vi "Main_24A.vi"() -> ()   [LabVIEW 2024]
uses:
  Cluster_Function.ctl
  ENUM_Operand.ctl
  <vilib>/Utility/error.llb/Trim Whitespace One-Sided.vi
panel:
  out "Answer Array":bool[](array[boolean])
  out "Map Final":map{string, bool}(c390)
  out "Wire Count":i32
  out "Array":T1[](array[typedef])
  out "Map Start":map{string, bool}(c390)
  in  "Select Data":enum32{"Example", "Example 2", "Puzzle"}(tab)
  in  "Example":string="x00: 1\nx01: 1\nx02: 1\ny00: 0\ny01: 1\ny02: 0\n\nx00 AND y00 -> z00\nx01 XOR y01 -> z01\nx02 OR y02 -> z02"
  in  "Example 2":string="x00: 1\nx01: 0\nx02: 1\nx03: 1\nx04: 0\ny00: 1\ny01: 1\ny02: 1\ny03: 1\ny04: 1\n\nntg XOR fgs -> mjb\ny02 OR x01 -> tnw\nkwq OR kpj -> z05\nx00 OR x03 -> fst\ntgd XOR rvg -> z01\nvdt OR tnw -> bfw\nbfw AND frj -> z10\nffh OR nrd -> bqk\ny00 AND y03 -> djm\ny03 OR y00 -> psh\nbqk OR frj -> z08\ntnw OR fst -> frj\ngnj AND tgd -> z11\nbfw XOR mjb -> z00\nx03 OR x00 -> vdt\ngnj AND wpb -> z02\nx04 AND y00 -> kjc\ndjm OR pbm -> qhw\nnrd AND vdt -> hwm\nkjc AND fst -> rvg\ny04 OR y02 -> fgs\ny01 AND x02 -> pbm\nntg OR kjc -> kwq\npsh XOR fgs -> tgd\nqhw XOR tgd -> z09\npbm OR djm -> kpj\nx03 XOR y03 -> ffh\nx00 XOR y04 -> ntg\nbfw OR bqk -> z06\nnrd XOR fgs -> wpb\nfrj XOR qhw -> z04\nbqk OR frj -> z07\ny03 OR x01 -> nrd\nhwm AND bqk -> z03\ntgd XOR rvg -> z12\ntnw OR pbm -> gnj"
  in  "Puzzle":string="x00: 1\nx01: 0\nx02: 1\nx03: 1\nx04: 0\nx05: 0\nx06: 1\nx07: 1\nx08: 0\nx09: 1\nx10: 1\nx11: 1\nx12: 1\nx13: 1\nx14: 1\nx15: 0\nx16: 1\nx17: 0\nx18: 1\nx19: 1\nx20: 0\nx21: 0\nx22: 1\nx23: 0\nx24: 1\nx25: 0\nx26: 1\nx27: 0\nx28: 1\nx29: 1\nx30: 0\nx31: 0\nx32: 1\nx33: 1\nx34: 1\nx35: 0\nx36: 1\nx37: 1\nx38: 0\nx39: 0\nx40: 1\nx41: 1\nx42: 0\nx43: 0\nx44: 1\ny00: 1\ny01: 0\ny02: 0\ny03: 1\ny04: 1\ny05: 0\ny06: 0\ny07: 0\ny08: 0\ny09: 0\ny10: 0\ny11: 1\ny12: 0\ny13: 0\ny14: 1\ny15: 1\ny16: 0\ny17: 0\ny18: 1\ny19: 0\ny20: 0\ny21: 0\ny22: 1\ny23: 1\ny24: 0\ny25: 0\ny26: 0\ny27: 1\ny28: 1\ny29: 1\ny30: 0\ny31: 1\ny32: 1\ny33: 0\ny34: 1\ny35: 1\ny36: 0\ny37: 0\ny38: 1\ny39: 1\ny40: 1\ny41: 0\ny42: 0\ny43: 1\ny44: 1\n\nnjs AND pvb -> fjh\ny12 AND x12 -> dcm\nsrv XOR dfc -> z22\nqwb XOR vmp -> z14\nnjs XOR pvb -> z10\ncjn OR dfj -> fgc\nkpp XOR tvh -> z34\ntbq OR rdf -> frv\ny40 AND x40 -> drs\npqh XOR mmh -> z05\nx26 XOR y26 -> jkt\nqqp AND dmw -> kqp\nqsh OR wfw -> qcr\nhvw AND qnn -> vgk\nbkc OR wsq -> ckv\nckv XOR bbh -> z03\nfrj XOR hqq -> z02\nqff OR stw -> wsv\nqpq XOR vnr -> z30\npbk XOR kqc -> z15\nmvp OR pbv -> dbj\nx15 AND y15 -> qsh\nwcs OR cqk -> kpp\nbmr XOR fgc -> z32\ny42 XOR x42 -> qjf\nsrv AND dfc -> rng\nrsq AND nts -> brq\nfhv AND hjw -> wwg\nx06 AND y06 -> phw\nvtf AND gdw -> kpc\nwvv AND wbf -> qdh\ny28 AND x28 -> nhs\ny04 AND x04 -> ttv\ncts XOR bcd -> qqp\nmmh AND pqh -> rkt\nhjw XOR fhv -> z37\njdd AND rbm -> z36\ndrt XOR tpt -> z31\ny20 XOR x20 -> gcf\nx27 AND y27 -> ptf\nqnn XOR hvw -> z41\nx13 AND y13 -> msq\ncbr XOR hjd -> z07\nmkv OR hgp -> z45\ny35 XOR x35 -> spp\nx08 XOR y08 -> nrk\ny03 XOR x03 -> bbh\nfhc OR ggh -> fwt\nwhj AND vrh -> qpj\nx34 XOR y34 -> tvh\ny43 AND x43 -> mpm\ny15 XOR x15 -> pbk\nx23 XOR y23 -> bcd\nbwv AND tcd -> sgv\nbcd AND cts -> jcd\nggs OR qmw -> tpt\ngdm XOR jkm -> z09\ny38 XOR x38 -> pgm\nx19 AND y19 -> vmc\ndtc OR ggg -> kqc\nhqq AND frj -> bkc\nsmv OR wwg -> bhh\ny17 AND x17 -> tfq\nx14 AND y14 -> dtc\ny39 AND x39 -> ggh\njmh AND cjc -> gfp\nmgj XOR wsv -> z12\nftd AND wcw -> hjm\ny19 XOR x19 -> whj\nnrk AND ksd -> vwf\nfgq AND spp -> drp\nrsq XOR nts -> z18\ny10 XOR x10 -> njs\nfrv XOR qdb -> z04\nwbk OR fcv -> fgq\nwhj XOR vrh -> z19\ntvh AND kpp -> wbk\ny39 XOR x39 -> pwt\nscg OR gkj -> grv\ndfn XOR qcr -> pbv\nx27 XOR y27 -> ftd\nsvg OR tfq -> rsq\nfkd XOR fwt -> z40\nx07 AND y07 -> pdq\ny13 XOR x13 -> hnt\ngrv XOR vpm -> z21\ny02 XOR x02 -> frj\njkt XOR dbp -> z26\nwdr OR jcd -> z23\nx21 AND y21 -> wns\ny08 AND x08 -> btn\nqqp XOR dmw -> z24\nx01 AND y01 -> wqt\nfrw AND hdp -> hgq\nfrk AND wpk -> hgp\nx07 XOR y07 -> cbr\nx29 AND y29 -> jgm\nsgv OR wqt -> hqq\ntpt AND drt -> dfj\nsdn OR rkt -> kqk\nfrv AND qdb -> vjj\nfjh OR thp -> ncw\ny26 AND x26 -> vvr\nx25 AND y25 -> kcs\nftd XOR wcw -> z27\ntcd XOR bwv -> z01\nbrk XOR kqk -> z06\nx10 AND y10 -> thp\nfrw XOR hdp -> z25\npgm AND bhh -> hsh\nx24 XOR y24 -> dmw\nvmc OR qpj -> bkv\nx44 AND y44 -> mkv\nknh OR vgk -> rps\ndfn AND qcr -> mvp\ntqj OR rng -> cts\ntbb OR wns -> srv\nmsq OR pjj -> vmp\ndrs OR ghn -> hvw\nhsh OR rrb -> rms\ndbj XOR bgt -> z17\nmpm OR kpc -> frk\nbgt AND dbj -> svg\nx40 XOR y40 -> fkd\nx16 AND y16 -> z16\ncbr AND hjd -> dvs\nfsb OR drv -> gdw\ncjc XOR jmh -> z29\npdq OR dvs -> ksd\nrpw OR fbq -> fhv\ny05 XOR x05 -> pqh\nx30 AND y30 -> ggs\nbmb OR drp -> jdd\nhnt XOR fbm -> z13\ny42 AND x42 -> fsb\nqpq AND vnr -> qmw\nx11 XOR y11 -> qff\ngcf AND bkv -> gkj\nwvv XOR wbf -> z28\nx05 AND y05 -> sdn\npqp OR phw -> hjd\njdd XOR rbm -> fbq\nnjt OR kqp -> frw\ny00 XOR x00 -> z00\ny31 AND x31 -> cjn\nx32 XOR y32 -> bmr\nx34 AND y34 -> fcv\ny24 AND x24 -> njt\ny06 XOR x06 -> brk\nx12 XOR y12 -> mgj\nckv AND bbh -> tbq\nrps XOR qjf -> z42\nx33 AND y33 -> cqk\ny09 AND x09 -> nhk\ny33 XOR x33 -> mbp\nx04 XOR y04 -> qdb\nx22 AND y22 -> tqj\ny20 AND x20 -> scg\ny01 XOR x01 -> tcd\nfgc AND bmr -> shp\nmbp XOR pnw -> z33\nfrk XOR wpk -> z44\ny43 XOR x43 -> vtf\nx37 XOR y37 -> hjw\ny03 AND x03 -> rdf\nrms XOR pwt -> z39\nbhh XOR pgm -> z38\nspp XOR fgq -> z35\ny22 XOR x22 -> dfc\nqjf AND rps -> drv\nkcs OR hgq -> dbp\ny29 XOR x29 -> cjc\nx25 XOR y25 -> hdp\nhbq OR dcm -> fbm\nbrk AND kqk -> pqp\nqwb AND vmp -> ggg\ngpb OR shp -> pnw\ny02 AND x02 -> wsq\nptf OR hjm -> wvv\nx18 XOR y18 -> nts\nx23 AND y23 -> wdr\nx09 XOR y09 -> jkm\nx36 AND y36 -> rpw\nx32 AND y32 -> gpb\nmbp AND pnw -> wcs\njgm OR gfp -> qpq\nx11 AND y11 -> qnw\nbkv XOR gcf -> z20\nnhk OR ftf -> pvb\ngdw XOR vtf -> z43\nvjj OR ttv -> mmh\nx41 AND y41 -> knh\nncw XOR qnw -> z11\ny28 XOR x28 -> wbf\ny36 XOR x36 -> rbm\nmgj AND wsv -> hbq\nhnt AND fbm -> pjj\nbrq OR bfd -> vrh\nx17 XOR y17 -> bgt\nksd XOR nrk -> z08\nx38 AND y38 -> rrb\nfwt AND fkd -> ghn\nncw AND qnw -> stw\nx18 AND y18 -> bfd\ny00 AND x00 -> bwv\ngdm AND jkm -> ftf\nrms AND pwt -> fhc\nx16 XOR y16 -> dfn\ny37 AND x37 -> smv\nx35 AND y35 -> bmb\ny30 XOR x30 -> vnr\njkt AND dbp -> dbt\ny41 XOR x41 -> qnn\nx31 XOR y31 -> drt\nqdh OR nhs -> jmh\nvwf OR btn -> gdm\ny44 XOR x44 -> wpk\nx14 XOR y14 -> qwb\nx21 XOR y21 -> vpm\npbk AND kqc -> wfw\nvvr OR dbt -> wcw\ngrv AND vpm -> tbb"
  out "Answer 49430469426918":u64
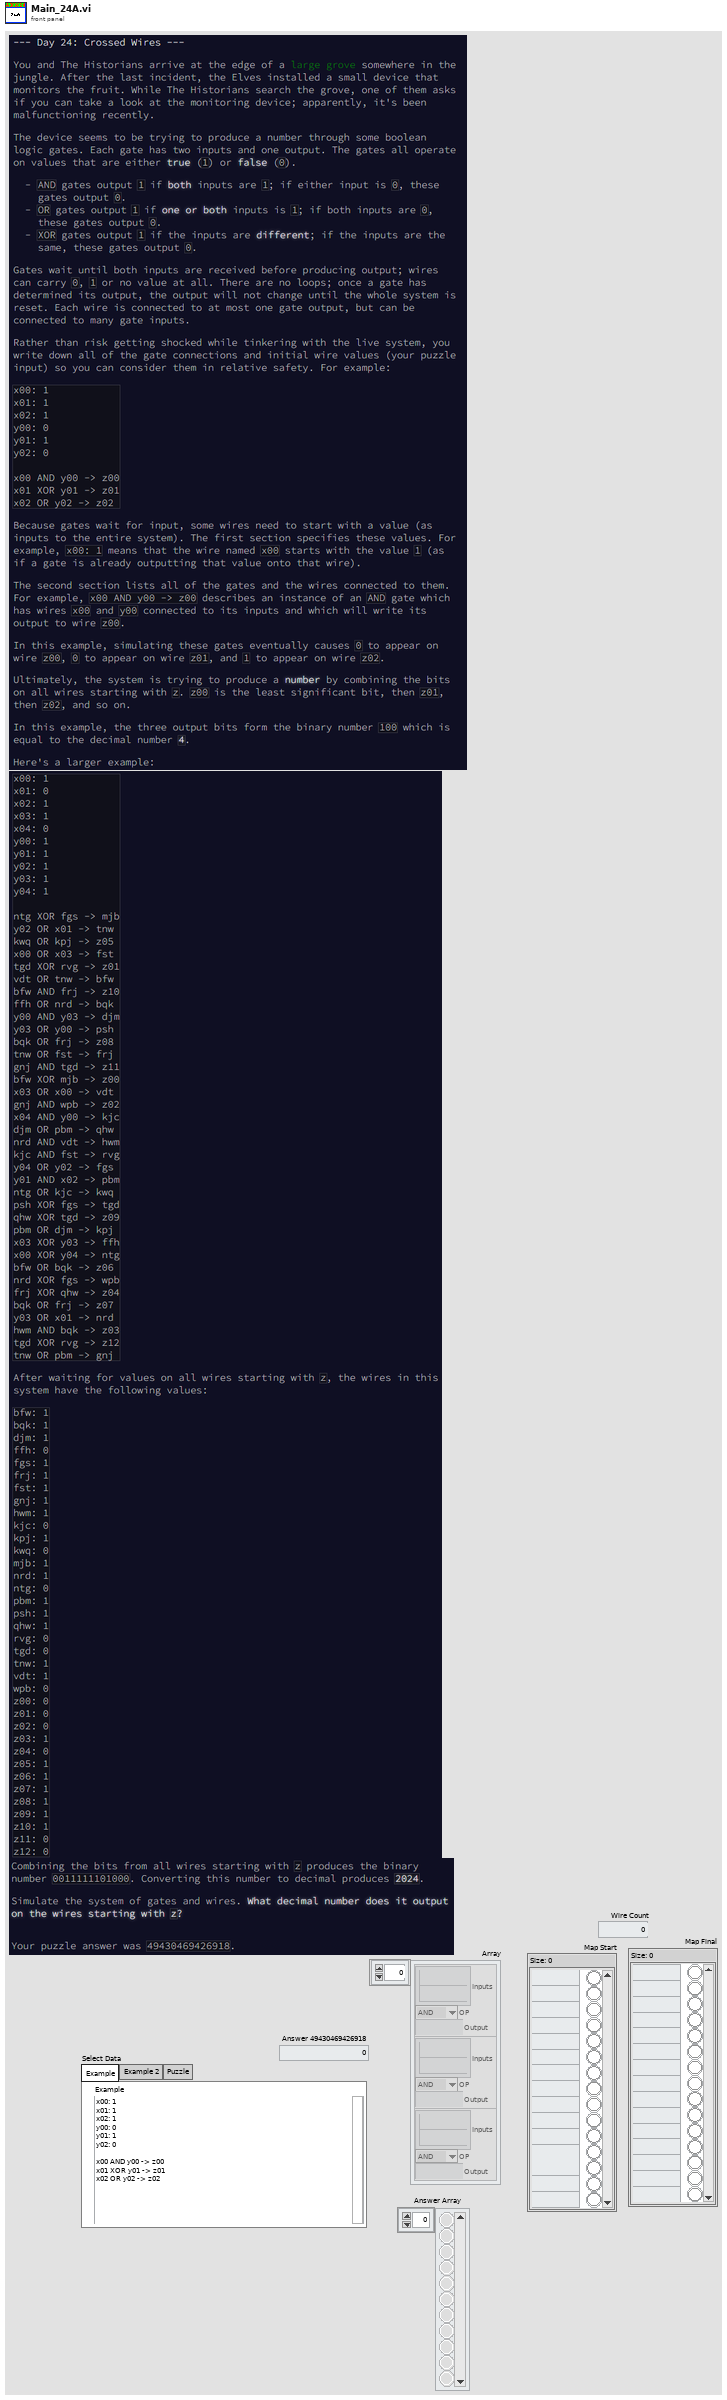
[diagram p1: front panel]
types:
  T1 = typedef "Cluster_Function.ctl" = cluster{"Inputs":string[], "OP":T2, "Output":string}
  T2 = typedef "ENUM_Operand.ctl" = enum16{"AND", "OR", "XOR"}
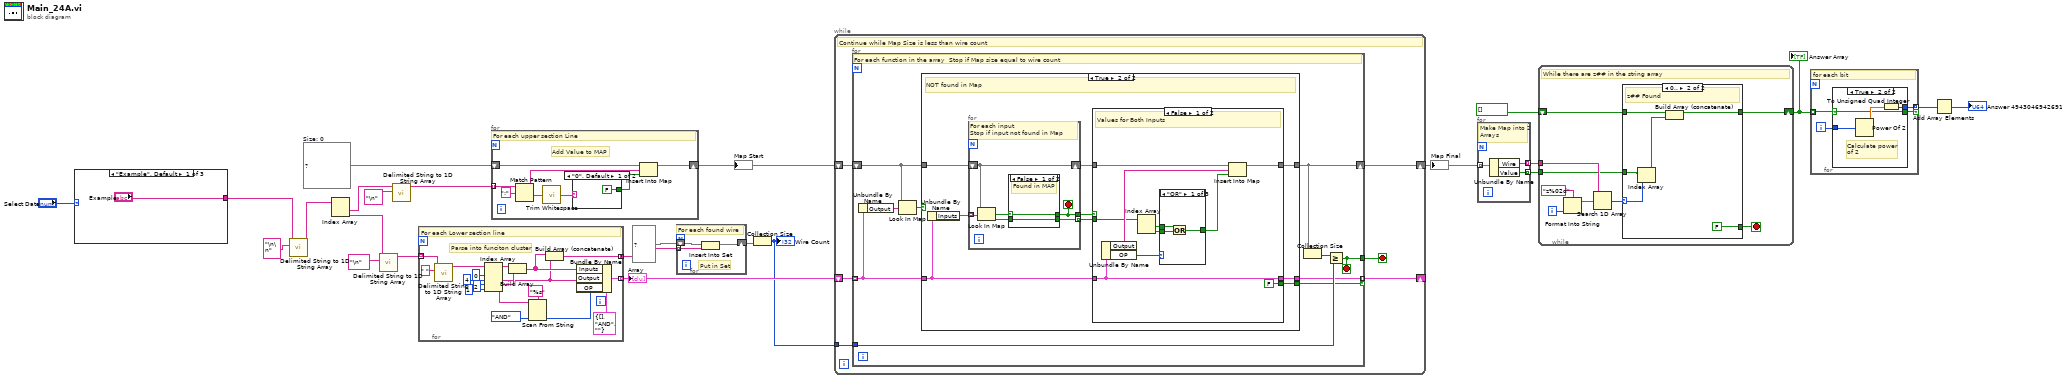
[diagram p0: block diagram]
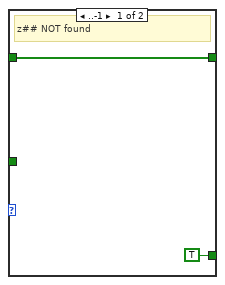
[diagram p3: hidden frame]
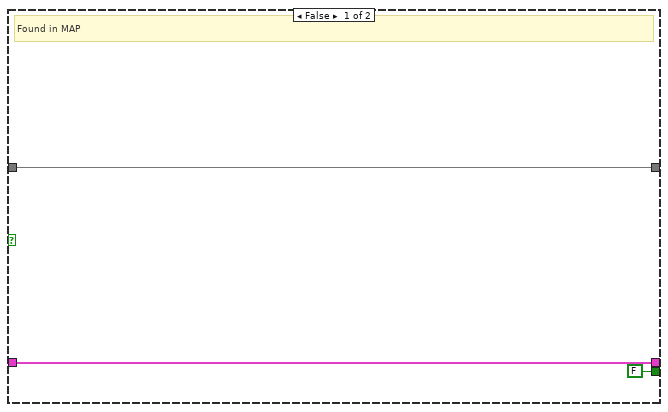
[diagram p4: hidden frame]
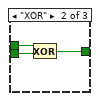
[diagram p5: hidden frame]
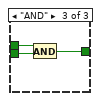
[diagram p6: hidden frame]
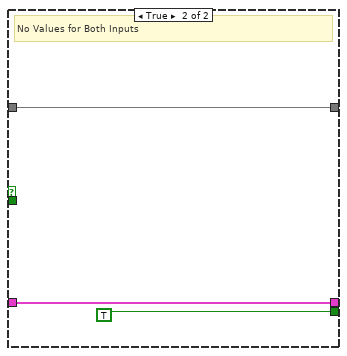
[diagram p7: hidden frame]
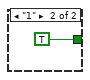
[diagram p9: hidden frame]
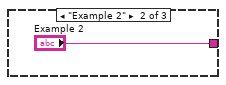
[diagram p10: hidden frame]
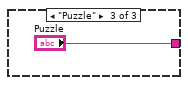
[diagram p11: hidden frame]
diagram:
  w17 = map{string, bool} {}  # Size: 0
  n1 = case shown="\"Example\", Default" "Select Data" {
    tunnel: ["Example" "Example 2" "Puzzle"] -> w22
    frame "Example", Default {
    }
    frame "Example 2" {
    }
    frame "Puzzle" {
    }
  }
  n2 = call <vilib>:"Delimited String to 1D String Array.vi"("delimiter"="\n\n" ("delimiter (Tab)"), "delimited string"=w22) -> ("string array"=w21:string[])  [unwired: 9 in]
  n3 = Index Array(array=w21) -> (element #1=w20:string, element #2=w16:string)  [unwired: 2 in]
  n4 = call <vilib>:"Delimited String to 1D String Array.vi"("delimiter"="\n" ("delimiter (Tab)"), "delimited string"=w16) -> ("string array"=w14:string[])  [unwired: 9 in]
  n5 = call <vilib>:"Delimited String to 1D String Array.vi"("delimiter"="\n" ("delimiter (Tab)"), "delimited string"=w20) -> ("string array"=w18:string[])  [unwired: 9 in]
  n6 = for {
    tunnel: w14 -> [w45] mode=indexing
    tunnel: [w31] -> w10 mode=indexing
    tunnel: [w28] -> w13 mode=concatenating
    # "Parse into funciton cluster"
    # "For each Lower section line"
    n7 = call <vilib>:"Delimited String to 1D String Array.vi"("delimiter"=" ", "delimited string"=w45) -> ("string array"=w43:string[])  [unwired: 9 in]
    n8 = Index Array(array=w43, index #1=0 ("index"), index #2=4 ("index"), index #3=2 ("index"), index #4=1 ("index")) -> (element #1=w38:string, element #2=w29:string, element #3=w37:string, element #4=w35:string)
    n9 = Build Array(w38, w37) -> (w30:string[])
    n10 = Scan From String(format string="%s", input string=w35, default 1=ENUM_Operand."AND" ("OP")) -> (output 1=w32:T2)  [unwired: 2 in, 3 out]
    n11 = Build Array (concatenate)(w30, w29) -> (w28:string[])
    n12 = Bundle By Name(cluster=T1 {"Inputs"=[], "OP"=enum."AND", "Output"=""} ("Function"), "Inputs"=w30, "Output"=w29, "OP"=w32) -> (w31:T1)
  }
  "Array" <- w10
  n13 = for {
    tunnel: w18 -> [w53] mode=indexing
    shift-right: [w50] -> w9
    shift-left: w17 -> [w51]
    # "Add Value to MAP"
    # "For each upper section Line"
    n14 = Match Pattern(string=w53, regular expression=":") -> (before substring=w49:string, after substring=w48:string)  [unwired: 1 in, 2 out]
    n15 = call <vilib>:"Trim Whitespace.vi"("string"=w48) -> ("trimmed string"=w47:string)  [unwired: 1 in]
    n16 = case shown="\"0\", Default" w47 {
      tunnel: [FALSE TRUE] -> w46
      frame "0", Default {
      }
      frame "1" {
      }
    }
    n17 = Insert Into Map(map in=w51, key=w49, value=w46) -> (map out=w50:map{string, bool})  [unwired: 2 out]
  }
  "Map Start" <- w9
  n18 = for {
    tunnel: w13 -> [w58] mode=indexing
    shift-right: [w56] -> w11
    shift-left: set{string} {} ("set in") -> [w57]
    # "Put in Set"
    # "For each found wire"
    n19 = Insert Into Set(10:w58, 11:w57) -> (3:w56:set{string})  [unwired: 1 out]
  }
  n20 = Collection Size(1:w11) -> (0:w8:i32)
  "Wire Count" <- w8
  n21 = while {
    shift-right: [w62] -> w7
    shift-left: w9 -> [w63]
    tunnel: w8 -> [w61]
    shift-right: [w59] -> _
    shift-left: w10 -> [w64]
    stop <- w60 stop-if-true
    # "Continue while Map Size is less than wire count"
    n22 = for {
      tunnel: w64 -> [w67] mode=indexing
      shift-right: [w71] -> w62
      shift-left: w63 -> [w72]
      tunnel: w61 -> [w69]
      tunnel: [w68] -> w60
      tunnel: [w66] -> w59 mode=indexing if=w65
      stop <- w68 stop-if-true
      # "For each function in the array  Stop if Map size equal to wire count"
      n23 = Unbundle By Name(w67) -> ("Output"=w74:string)
      n24 = Look In Map(map=w72, key=w74) -> (key not found?=w73:bool)  [unwired: 1 in, 1 out]
      n25 = case shown="True" w73 {
        tunnel: w72 -> [w77 w86]
        tunnel: [w77 w82] -> w71
        tunnel: w67 -> [w76 w81]
        tunnel: [w76 w80] -> w66
        tunnel: [FALSE w79] -> w65
        frame False {
          # "Found in MAP"
        }
        frame True {
          # "NOT found in Map"
          n26 = Unbundle By Name(w81) -> ("Inputs"=w85:string[])
          n27 = for {
            shift-right: [w113] -> w84
            shift-left: w86 -> [w113]
            tunnel: w85 -> [w114] mode=indexing
            tunnel: [w111] -> w78 mode=indexing
            tunnel: [w109] -> w83
            stop <- w109 stop-if-true
            # "For each input\nStop if input not found in Map"
            n28 = Look In Map(map=w113, key=w114) -> (key not found?=w112:bool, value=w110:bool)  [unwired: 1 in]
            n29 = case shown="False" w112 {
              selector: w112 -> [w116 w117]
              tunnel: [w116 w117] -> w109
              tunnel: [w115 _] -> w111
              tunnel: w110 -> [w115 _]
              frame False {
                # "Found in MAP"
              }
              frame True {
                # "NOT Found in Map"
              }
            }
          }
          n30 = case shown="False" w83 {
            tunnel: w84 -> [w94 w108]
            tunnel: [w93 w108] -> w82
            tunnel: w81 -> [w95 w107]
            tunnel: [w95 w107] -> w80
            tunnel: [FALSE TRUE] -> w79
            tunnel: w78 -> [w90 _]
            frame False {
              # "Values for Both Inputs"
              n31 = Unbundle By Name(w95) -> ("Output"=w92:string, "OP"=w91:T2)
              n32 = Index Array(array=w90) -> (element #1=w89:bool, element #2=w88:bool)  [unwired: 2 in]
              n33 = case shown="\"OR\"" w91 {
                tunnel: w89 -> [w99 w102 w105]
                tunnel: w88 -> [w98 w101 w104]
                tunnel: [w97 w100 w103] -> w87
                frame "OR" {
                  n34 = Or(x=w99, y=w98) -> (x .or. y?=w97:bool)
                }
                frame "XOR" {
                  n35 = Exclusive Or(1:w101, 2:w102) -> (0:w100:bool)
                }
                frame "AND" {
                  n36 = And(x=w105, y=w104) -> (x .and. y?=w103:bool)
                }
              }
              n37 = Insert Into Map(map in=w94, key=w92, value=w87) -> (map out=w93:map{string, bool})  [unwired: 2 out]
            }
            frame True {
              # "No Values for Both Inputs"
            }
          }
        }
      }
      n38 = Collection Size(1:w71) -> (0:w70:i32)
      n39 = Greater Or Equal?(x=w70, y=w69) -> (x >= y?=w68:bool)
    }
  }
  "Map Final" <- w7
  n40 = for {
    tunnel: w7 -> [w120] mode=indexing
    tunnel: [w119] -> w6 mode=indexing
    tunnel: [w118] -> w5 mode=indexing
    # "Make Map into 2 Arrays"
    n41 = Unbundle By Name(w120) -> ("Wire"=w119:string, "Value"=w118:bool)
  }
  n42 = while {
    tunnel: w6 -> [w127]
    tunnel: w5 -> [w121]
    shift-right: [w122] -> w3
    shift-left: bool[] [] -> [w124]
    i -> [w129]
    stop <- w123 stop-if-true
    # "While there are z## in the string array"
    n43 = Format Into String(format string="z%02d", w129) -> (resulting string=w126:string)  [unwired: 2 in, 1 out]
    n44 = Search 1D Array(1D array=w127, element=w126) -> (index of element=w125:i32)  [unwired: 1 in]
    n45 = case shown="0.." w125 {
      selector: w125 -> [_ w133]
      tunnel: w124 -> [w131 w136]
      tunnel: [TRUE FALSE] -> w123
      tunnel: [w131 w135] -> w122
      tunnel: w121 -> [_ w134]
      frame ..-1 {
        # "z## NOT found"
      }
      frame 0.. {
        # "z## Found"
        n46 = Index Array(array=w134, index=w133) -> (element=w132:bool)
        n47 = Build Array (concatenate)(w136, w132) -> (w135:bool[])
      }
    }
  }
  "Answer Array" <- w3
  n48 = for {
    tunnel: w3 -> [w140] mode=indexing
    tunnel: [w139] -> w2 mode=indexing if=w138
    i -> [w141]
    # "for each bit"
    n49 = case shown="True" w140 {
      selector: w140 -> [w142 w144]
      tunnel: w141 -> [_ w146]
      tunnel: [w142 w144] -> w138
      tunnel: [_ w143] -> w139
      frame False {
      }
      frame True {
        # "Calculate power\nof 2"
        n50 = Power Of 2(x=w146) -> (2^x=w145:dbl)
        n51 = To Unsigned Quad Integer(1:w145) -> (0:w143:u64)
      }
    }
  }
  n52 = Add Array Elements(numeric array=w2) -> (sum=→"Answer 49430469426918":u64)
